vi "采配水通讯指令.vi"(10 "数据":variant, 11 "命令":T1(ring)) -> ()   [LabVIEW 2016, in "PLC.lvlib"]
uses:
  PLC.lvlib
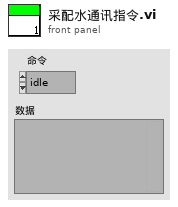
[diagram p1: front panel]
types:
  T1 = enum16{"idle", "init", "读状态", "读参数", "多个写入", "单个写入", "线圈写入"}
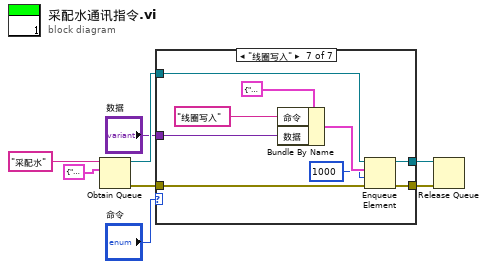
[diagram p0: block diagram]
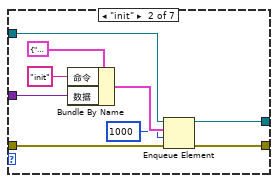
[diagram p3: hidden frame]
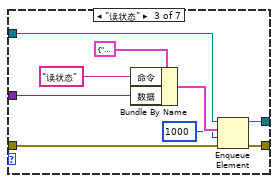
[diagram p4: hidden frame]
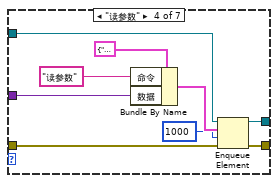
[diagram p5: hidden frame]
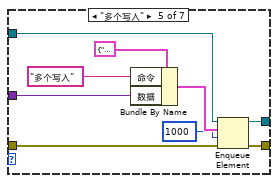
[diagram p6: hidden frame]
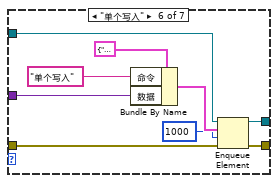
[diagram p7: hidden frame]
diagram:
  n1 = Obtain Queue(name (unnamed)="采配水" ("名称（未命名）"), element data type=cluster{"命令":string, "数据":variant} {"命令"="", "数据"=variant}) -> (queue out=w6:refnum<queue>, error out=w5:errorcluster)  [unwired: 3 in, 1 out]
  n2 = case shown="\"线圈写入\"" "命令" {
    tunnel: w6 -> [w10 w19 w28 w37 w46 w55 w64]
    tunnel: w5 -> [w9 w18 w27 w36 w45 w54 w63]
    tunnel: [w10 w17 w26 w35 w44 w53 w62] -> w4
    tunnel: [w9 w16 w25 w34 w43 w52 w61] -> w3
    tunnel: "数据" -> [_ w14 w23 w32 w41 w50 w59]
    frame "idle", Default {
    }
    frame "init" {
      n3 = Bundle By Name(cluster=cluster{"命令":string, "数据":variant} {"命令"="", "数据"=variant}, "命令"="init", "数据"=w14) -> (w13:cluster{"命令":string, "数据":variant})
      n4 = Enqueue Element(queue=w19, element=w13, timeout in ms (-1)=1000 ("超时毫秒(-1)"), error in (no error)=w18) -> (queue out=w17:refnum<queue>, error out=w16:errorcluster)  [unwired: 1 out]
    }
    frame "读状态" {
      n5 = Bundle By Name(cluster=cluster{"命令":string, "数据":variant} {"命令"="", "数据"=variant}, "命令"="读状态", "数据"=w23) -> (w22:cluster{"命令":string, "数据":variant})
      n6 = Enqueue Element(queue=w28, element=w22, timeout in ms (-1)=1000 ("超时毫秒(-1)"), error in (no error)=w27) -> (queue out=w26:refnum<queue>, error out=w25:errorcluster)  [unwired: 1 out]
    }
    frame "读参数" {
      n7 = Bundle By Name(cluster=cluster{"命令":string, "数据":variant} {"命令"="", "数据"=variant}, "命令"="读参数", "数据"=w32) -> (w31:cluster{"命令":string, "数据":variant})
      n8 = Enqueue Element(queue=w37, element=w31, timeout in ms (-1)=1000 ("超时毫秒(-1)"), error in (no error)=w36) -> (queue out=w35:refnum<queue>, error out=w34:errorcluster)  [unwired: 1 out]
    }
    frame "多个写入" {
      n9 = Bundle By Name(cluster=cluster{"命令":string, "数据":variant} {"命令"="", "数据"=variant}, "命令"="多个写入", "数据"=w41) -> (w40:cluster{"命令":string, "数据":variant})
      n10 = Enqueue Element(queue=w46, element=w40, timeout in ms (-1)=1000 ("超时毫秒(-1)"), error in (no error)=w45) -> (queue out=w44:refnum<queue>, error out=w43:errorcluster)  [unwired: 1 out]
    }
    frame "单个写入" {
      n11 = Bundle By Name(cluster=cluster{"命令":string, "数据":variant} {"命令"="", "数据"=variant}, "命令"="单个写入", "数据"=w50) -> (w49:cluster{"命令":string, "数据":variant})
      n12 = Enqueue Element(queue=w55, element=w49, timeout in ms (-1)=1000 ("超时毫秒(-1)"), error in (no error)=w54) -> (queue out=w53:refnum<queue>, error out=w52:errorcluster)  [unwired: 1 out]
    }
    frame "线圈写入" {
      n13 = Bundle By Name(cluster=cluster{"命令":string, "数据":variant} {"命令"="", "数据"=variant}, "命令"="线圈写入", "数据"=w59) -> (w58:cluster{"命令":string, "数据":variant})
      n14 = Enqueue Element(queue=w64, element=w58, timeout in ms (-1)=1000 ("超时毫秒(-1)"), error in (no error)=w63) -> (queue out=w62:refnum<queue>, error out=w61:errorcluster)  [unwired: 1 out]
    }
  }
  n15 = Release Queue(queue=w4, error in (no error)=w3) -> ()  [unwired: 1 in, 3 out]
